vi "Call VI.vi"(8 "error in":errorcluster, 9 "DVR":refnum<data-value>, 10 "section":string, 11 "Low Speed in":refnum<class "Low Speed.lvclass">) -> (0 "error out":errorcluster, 1 "VI Ref":refnum<vi>, 2 "Asynch Ref":refnum<vi>, 3 "Low Speed out":refnum<class "Low Speed.lvclass">)   [LabVIEW 2020, in "Low Speed.lvclass"]
uses:
  Low Speed.lvclass
  Parent Class/Speed Mode/Speed Mode.lvclass
  SubVIs/Lowspeed Mode.vi
  Low Speed.lvclass/Low Speed.ctl
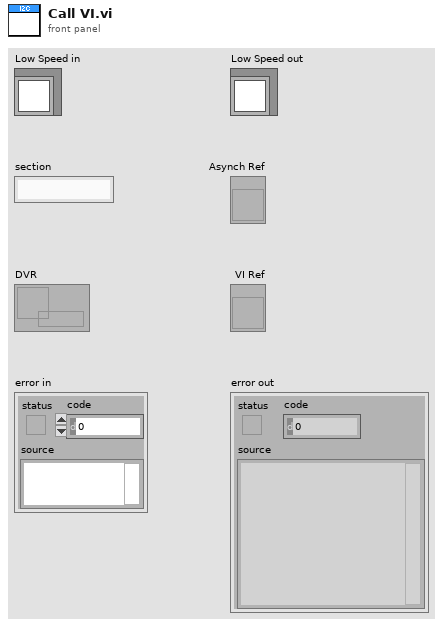
[diagram p1: front panel]
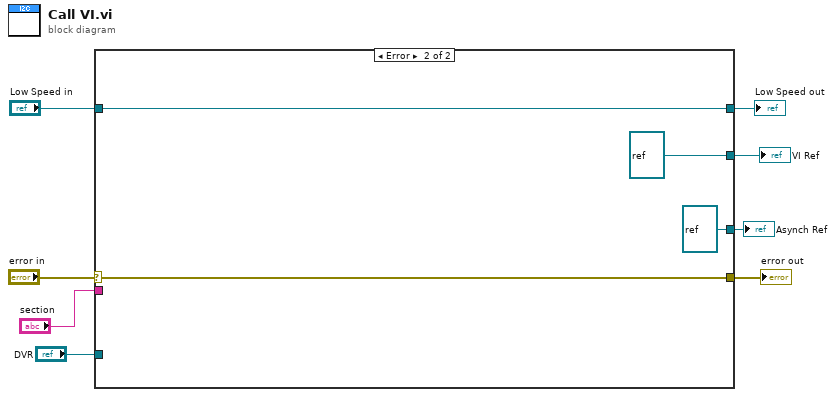
[diagram p0: block diagram]
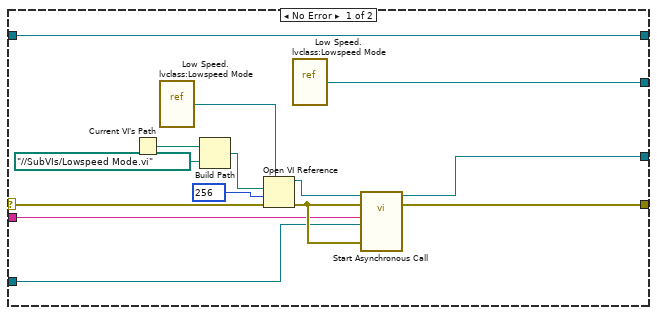
[diagram p2: hidden frame]
diagram:
  n1 = case shown="Error" "error in" {
    selector: "error in" -> [w17 w26]
    tunnel: [w21 w26] -> w7
    tunnel: [w22 w25] -> w5
    tunnel: "Low Speed in" -> [w22 w25]
    tunnel: "section" -> [w11 _]
    tunnel: [w20 refnum<vi> refnum] -> w3
    tunnel: "DVR" -> [w10 _]
    tunnel: [w9 refnum<vi> refnum] -> w1
    frame No Error {
      n2 = Current VI's Path() -> (path=w19:path)
      n3 = vi-ref "Low Speed.lvclass:Lowspeed Mode.vi"() -> (w13:refnum<vi>)
      n4 = Build Path(base path=w19, name or relative path=path "../../SubVIs/Lowspeed Mode.vi") -> (appended path=w16:path)
      n5 = Open VI Reference(type specifier VI Refnum (for type only)=w13, vi path=w16, options=256, error in (no error)=w17) -> (vi reference=w12:refnum<vi>, error out=w14:errorcluster)  [unwired: 2 in]
      n6 = vi-ref "Low Speed.lvclass:Lowspeed Mode.vi"() -> (w20:refnum<vi>)
      n7 = call-by-ref "Start Asynchronous Call"(reference=w12, error in=w14, "section"=w11, "DVR"=w10, "error in"=w14) -> (reference out=w9:refnum<vi>, error out=w21:errorcluster)  [unwired: 11 in, 2 out]
    }
    frame Error {
    }
  }
  "error out" <- w7
  "Low Speed out" <- w5
  "VI Ref" <- w3
  "Asynch Ref" <- w1
